vi "Set Cells (2D String).vi"(7 "Values":string[][](array[string]), 8 "error in (no error)":errorcluster, 9 "Column (0)":i32, 10 "Row (0)":i32, 11 "Excel Legacy in":refnum<class "Excel Legacy.lvclass">) -> (0 "error out":errorcluster, 3 "Excel Legacy out":refnum<class "Excel Legacy.lvclass">)   [LabVIEW 2013, in "Excel Legacy.lvclass"]
uses:
  Excel Legacy.lvclass
  Spreadsheet.lvclass
  Excel Legacy.lvclass/Excel Legacy.ctl
  C:/PhaeronGit/LVNPOI/Resources/NPOI 2.1.1 dotnet2/NPOI.dll
  Resources/NPOI 2.1.1 dotnet2/NPOI.dll
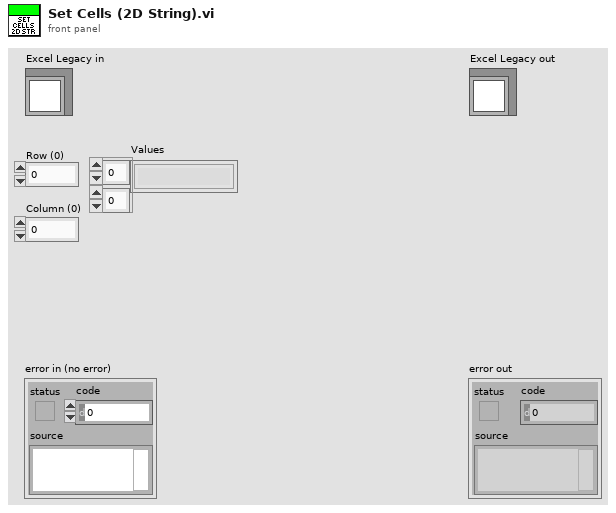
[diagram p1: front panel]
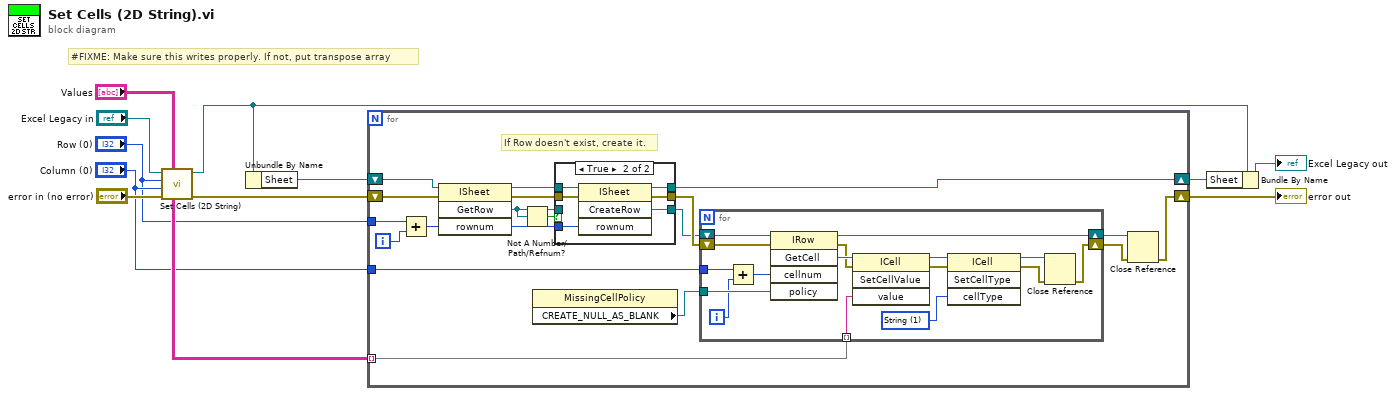
[diagram p0: block diagram]
diagram:
  # "#FIXME: Make sure this writes properly. If not, put transpose array"
  n1 = call-parent "Set Cells (2D String).vi"("Values"="Values", "error in (no error)"="error in (no error)", "Column (0)"="Column (0)", "Row (0)"="Row (0)", "Spreadsheet in"="Excel Legacy in") -> ("error out"=w9:errorcluster, "Spreadsheet out"=w2:refnum<class "Excel Legacy.lvclass">)  [unwired: 5 in]
  n2 = Unbundle By Name(w2) -> ("Sheet"=w1:refnum<k24>)
  n3 = for {
    tunnel: "Column (0)" -> [w28]
    tunnel: "Row (0)" -> [w19]
    shift-right: [w18] -> w3
    shift-left: w1 -> [w20]
    shift-right: [w26] -> w5
    shift-left: w9 -> [w21]
    tunnel: "Values" -> [w14] mode=indexing
    i -> [w12]
    # "If Row doesn't exist, create it."
    n4 = Add(x=w19, y=w12) -> (x+y=w13:i32)
    n5 = invoke class="ISheet" method="GetRow"(reference=w20, error in=w21, "rownum"=w13) -> (reference out=w22:refnum<k24>, error out=w23:errorcluster, "GetRow"=w25:refnum<k24>)  [unwired: 1 in, 1 out]
    n6 = Not A Number/Path/Refnum?(number/path/refnum=w25) -> (NaN/Path/Refnum?=w24:bool)
    n7 = property class="MissingCellPolicy"() -> ("CREATE_NULL_AS_BLANK"=w15:refnum<k24>)  [unwired: 2 in, 2 out]
    n8 = case shown="True" w24 {
      tunnel: w22 -> [w48 w54]
      tunnel: w23 -> [w47 w53]
      tunnel: [w47 w52] -> w17
      tunnel: [w48 w51] -> w18
      tunnel: w13 -> [_ w50]
      tunnel: [w46 w49] -> w16
      tunnel: w25 -> [w46 _]
      frame False {
      }
      frame True {
        n9 = invoke class="ISheet" method="CreateRow"(reference=w54, error in=w53, "rownum"=w50) -> (reference out=w51:refnum<k24>, error out=w52:errorcluster, "CreateRow"=w49:refnum<k24>)  [unwired: 1 in, 1 out]
      }
    }
    n10 = for {
      tunnel: w28 -> [w44]
      tunnel: w15 -> [w38]
      shift-right: [w45] -> w29
      shift-left: w16 -> [w39]
      shift-right: [w41] -> w27
      shift-left: w17 -> [w40]
      tunnel: w14 -> [w30] mode=indexing
      i -> [w36]
      w31 = 1 items=["Numeric"=0, "String"=1, "Formula"=2, "Blank"=3, "Boolean"=4, "Error"=5, "Unknown"=-1] ("cellType")
      n11 = Add(x=w44, y=w36) -> (x+y=w37:i32)
      n12 = invoke class="IRow" method="GetCell"(reference=w39, error in=w40, "cellnum"=w37, "policy"=w38) -> (reference out=w45:refnum<k24>, error out=w42:errorcluster, "GetCell"=w43:refnum<k24>)  [unwired: 1 in, 2 out]
      n13 = invoke class="ICell" method="SetCellValue"(reference=w43, error in=w42, "value"=w30) -> (reference out=w35:refnum<k24>, error out=w34:errorcluster)  [unwired: 1 in, 2 out]
      n14 = invoke class="ICell" method="SetCellType"(reference=w35, error in=w34, "cellType"=w31) -> (reference out=w33:refnum<k24>, error out=w32:errorcluster)  [unwired: 1 in, 2 out]
      n15 = Close Reference(reference=w33, error in (no error)=w32) -> (error out=w41:errorcluster)
    }
    n16 = Close Reference(reference=w29, error in (no error)=w27) -> (error out=w26:errorcluster)
  }
  "error out" <- w5
  n17 = Bundle By Name(cluster=w2, "Sheet"=w3) -> (→"Excel Legacy out":refnum<class "Excel Legacy.lvclass">)
